vi "ReCalculateCoincidence.vi"(0 "orig dim":cluster{"x":u32, "y":u32}, 1 "new dim":cluster{"x":u32, "y":u32}, 2 "threshold":u32, 3 "coincidence settings":T1 {"center peak (µs)" format="%.2f"; "length [µs]" format="%.2f"}, 4 "ratio":bool) -> (5 "output":dbl[][](array[numeric]) format="%.2f")   [LabVIEW 2009]
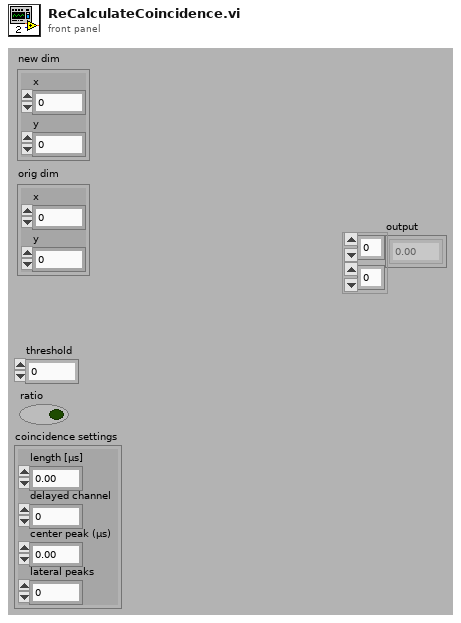
[diagram p1: front panel]
types:
  T1 = cluster{"length [µs]":dbl, "delayed channel":u8, "center peak (µs)":dbl, "lateral peaks":u32}
  T2 = cluster{"origin (ns)":dbl, "offset (ns)":dbl, "histogram":u32[]}[][]
  T3 = cluster{"origin (ns)":dbl, "offset (ns)":dbl, "histogram":u32[]}
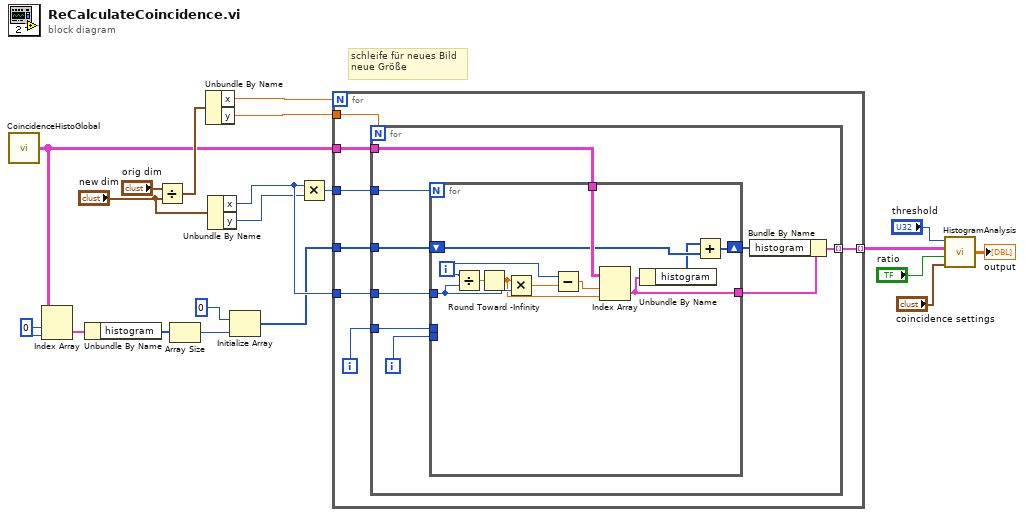
[diagram p0: block diagram]
diagram:
  w6 = 0 ("index (row)")
  # "schleife für neues Bild\nneue Größe"
  n1 = call "CoincidenceHistoGlobal.vi"() -> ("Array"=w7:T2)  [unwired: 2 in]
  n2 = Index Array(array=w7, index (row)=w6, index (col)=w6) -> (element=w5:T3)
  n3 = Unbundle By Name(w5) -> ("histogram"=w4:u32[])
  n4 = Divide(x="orig dim", y="new dim") -> (x/y=w19:cluster{"x":dbl, "y":dbl})
  n5 = Array Size(array=w4) -> (size(s)=w3:i32)
  n6 = Unbundle By Name(w19) -> ("x"=w12:dbl, "y"=w11:dbl)
  n7 = Unbundle By Name("new dim") -> ("x"=w9:u32, "y"=w8:u32)
  n8 = Initialize Array(u32 0 ("element"), w3) -> (w1:u32[])
  n9 = Multiply(x=w9, y=w8) -> (x*y=w18:u32)
  n10 = for {
    N: w12 -> [_]
    tunnel: w7 -> [w26]
    tunnel: w11 -> [w27]
    tunnel: w18 -> [w25]
    tunnel: w9 -> [w23]
    tunnel: [w22] -> w17 mode=indexing
    tunnel: w1 -> [w21]
    i -> [w24]
    n11 = for {
      N: w27 -> [_]
      tunnel: w26 -> [w34]
      tunnel: w25 -> [w36]
      tunnel: w24 -> [w35]
      tunnel: w23 -> [w32]
      tunnel: [w29] -> w22 mode=indexing
      tunnel: w21 -> [w28]
      i -> [w33]
      n12 = for {
        N: w36 -> [_]
        shift-right: [w45] -> w30
        shift-left: w28 -> [w46]
        tunnel: w35 -> [_]
        tunnel: w34 -> [w47]
        tunnel: w33 -> [_]
        tunnel: w32 -> [w43]
        tunnel: [w37] -> w31
        i -> [w41]
        n13 = Divide(x=w41, y=w43) -> (x/y=w44:dbl)
        n14 = Round Toward -Infinity(1:w44) -> (0:w40:dbl)
        n15 = Multiply(x=w40, y=w43) -> (x*y=w42:dbl)
        n16 = Subtract(x=w41, y=w42) -> (x-y=w39:dbl)
        n17 = Index Array(array=w47, index (row)=w39, index (col)=w40) -> (element=w37:T3)
        n18 = Unbundle By Name(w37) -> ("histogram"=w38:u32[])
        n19 = Add(x=w38, y=w46) -> (x+y=w45:u32[])
      }
      n20 = Bundle By Name(cluster=w31, "histogram"=w30) -> (w29:T3)
    }
  }
  n21 = call "HistogramAnalysis.vi"("coincidence settings"="coincidence settings", "ratio"="ratio", "Array 2"=w17, "threshold"="threshold") -> ("Array"=→"output":dbl[][])
